vi "InsertIntoDBSubVI.vi"(4 "Refnum in":T1, 5 "Data":dbl, 6 "Conexion":string, 7 "error in (no error)":errorcluster) -> (0 "Refnum out":T1, 3 "error out":errorcluster)   [LabVIEW 2016]
doc: "Takes two values, Name of Conection and Data, and inserts them into the data base indentified by the Refnum in"
uses:
  <vilib>/addons/database/Connection.llb/Conn ObjectReference.ctl
  <vilib>/addons/database/NI_Database_API.lvlib
panel:
  out "variant":variant
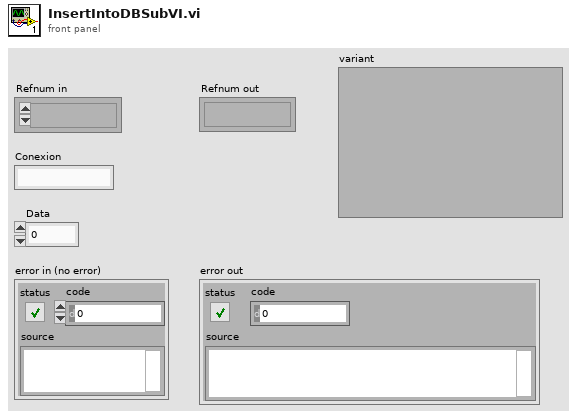
[diagram p1: front panel]
types:
  T1 = typedef "NI_Database_API.lvlib/Conn ObjectReference.ctl" = refnum<k1>
  T2 = cluster{"date/time string":string, "date/time string":string, "Conexion":string, "Data":dbl, dbl, dbl, dbl, string}
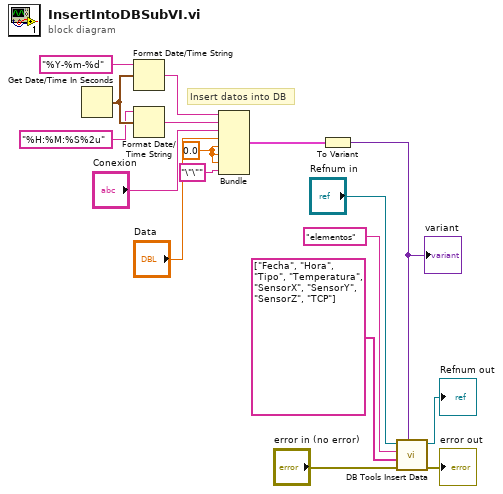
[diagram p0: block diagram]
diagram:
  w7 = 0.0
  # "Insert datos into DB"
  n1 = Get Date/Time In Seconds() -> (seconds since 1Jan1904=w12:timestamp)
  n2 = Format Date/Time String(time format string (%c)="%Y-%m-%d", seconds (now)=w12) -> (date/time string=w10:string)  [unwired: 1 in]
  n3 = Format Date/Time String(time format string (%c)="%H:%M:%S%2u", seconds (now)=w12) -> (date/time string=w13:string)  [unwired: 1 in]
  n4 = Bundle("date/time string"=w10, "date/time string"=w13, "Conexion"="Conexion", "Data"="Data", w7, w7, w7, "\"\"") -> (w11:T2)  [unwired: 1 in]
  n5 = To Variant(anything=w11) -> (Variant=w14:variant)
  "variant" <- w14
  n6 = call <vilib>:"DB Tools Insert Data.vi"("data"=w14, "error in (no error)"="error in (no error)", "columns"=string[] ["Fecha", "Hora", "Tipo", "Temperatura", "SensorX", "SensorY", "SensorZ", "TCP"], "table"="elementos", "connection reference"="Refnum in") -> ("error out"=→"error out":errorcluster, "connection reference out"=→"Refnum out":T1)  [unwired: 5 in]
